vi "INI to String Array.vi"(8 "Error IN":errorcluster, 10 "Section":string, 11 "Path":path) -> (0 "Error OUT":errorcluster, 3 "Array":string[][](array[string]))   [LabVIEW 2013]
uses:
  <vilib>/Utility/config.llb/Read Key (String).vi
  <vilib>/Utility/config.llb/NI_LVConfig.lvlib
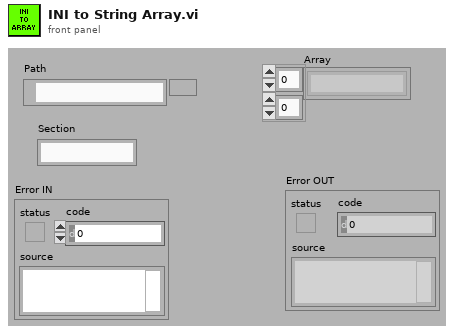
[diagram p1: front panel]
types:
  T1 = typedef "NI_LVConfig.lvlib/Config Data RefNum.ctl" = refnum<k1>
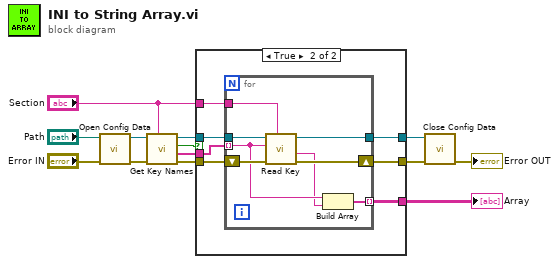
[diagram p0: block diagram]
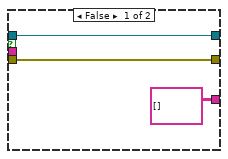
[diagram p2: hidden frame]
diagram:
  n1 = call <vilib>:"Open Config Data.vi"("error in (no error)"="Error IN", "configuration file path"="Path") -> ("error out"=w8:errorcluster, "refnum"=w6:T1)  [unwired: 7 in, 1 out]
  n2 = call <vilib>:"Get Key Names.vi"("section"="Section", "error in (no error)"=w8, "refnum"=w6) -> ("error out"=w7:errorcluster, "key names"=w4:string[], "section exists?"=w1:bool, "refnum out"=w5:T1)  [unwired: 5 in]
  n3 = case shown="True" w1 {
    tunnel: [w15 w23] -> w11
    tunnel: [w16 w22] -> w10
    tunnel: w7 -> [w15 w21]
    tunnel: w5 -> [w16 w20]
    tunnel: w4 -> [_ w19]
    tunnel: "Section" -> [_ w18]
    tunnel: [string[][] [] w17] -> w2
    frame False {
    }
    frame True {
      n4 = for {
        tunnel: w20 -> [w29]
        shift-right: [w30] -> w23
        shift-left: w21 -> [w31]
        tunnel: [w27] -> w22
        tunnel: w19 -> [w26] mode=indexing
        tunnel: w18 -> [w28]
        tunnel: [w24] -> w17 mode=indexing
        n5 = call-poly <vilib>:"Read Key.vi"("section"=w28, "error in (no error)"=w31, "key"=w26, "refnum"=w29) -> ("error out"=w30:errorcluster, "value"=w25:string, "refnum out"=w27:T1)  [unwired: 4 in, 1 out]
        n6 = Build Array(w26, w25) -> (w24:string[])
      }
    }
  }
  "Array" <- w2
  n7 = call <vilib>:"Close Config Data.vi"("error in (no error)"=w11, "refnum"=w10) -> ("error out"=→"Error OUT":errorcluster)  [unwired: 8 in, 1 out]
